vi "Load_Info.vi"(8 "error in (no error)":errorcluster, 11 "AB_RESTfulWebService in":refnum<class "AB_RESTfulWebService.lvclass">) -> (0 "error out":errorcluster, 3 "AB_RESTfulWebService out":refnum<class "AB_RESTfulWebService.lvclass">)   [LabVIEW 2020, in "AB_RESTfulWebService.lvclass"]
uses:
  <vilib>/AppBuilder/AB_Classes/RESTful/AB_RESTfulWebService.lvclass
  e:/builds/penguin/labview/branches/2020/dev/dist/vi.lib/AppBuilder/AB_Classes/Build/AB_Build.lvclass
  <vilib>/AppBuilder/AB_Classes/RESTful/AB_RESTfulWebService.ctl
  <vilib>/AppBuilder/AB_Classes/RESTful/AB_RESTful_RoutingTemplate.ctl
  <vilib>/AppBuilder/AB_Classes/RESTful/AB_RESTful_RoutingType.ctl
  <vilib>/AppBuilder/AB_Classes/RESTful/AB_RESTful_HTTPMethodType.ctl
  <vilib>/AppBuilder/AB_Classes/RESTful/AB_RESTful_ServiceAttribute.ctl
  <vilib>/AppBuilder/AB_Classes/RESTful/AB_RESTful_ServiceAttributeType.ctl
  <vilib>/AppBuilder/RW_Project/AB_RW_Project_PropBag_Action.ctl
  <vilib>/AppBuilder/AB_Classes/RESTful/AB_RESTfulWebService.lvclass/AB_RESTfulWebService.ctl
  <vilib>/AppBuilder/AB_Classes/WebService/AB_WebService.lvclass
  <vilib>/AppBuilder/AB_Classes/Build/AB_Build.lvclass
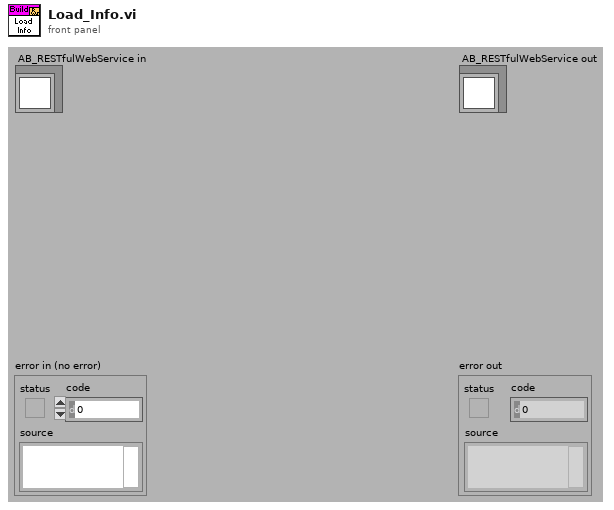
[diagram p1: front panel]
types:
  T1 = typedef "AB_RESTfulWebService.ctl" = cluster{"routing templates":T2[], "defaultStaticDoc":string, "eng_attributes":T5[], "Privilege Mapping":cluster{"Privilege":string, "Description":string, "Role":string}[]}
  T2 = typedef "AB_RESTful_RoutingTemplate.ctl" = cluster{"Template":string, "Routing Type":T3, "HTTP Method Type":T4, "VIName":string, "Default String":string, "Require API key":bool, "Auth permissions":string[], "eng_Static Alias":string, "Required Privilege":string}
  T3 = typedef "AB_RESTful_RoutingType.ctl" = enum32{"Method", "Static"}
  T4 = typedef "AB_RESTful_HTTPMethodType.ctl" = enum32{"GET", "POST", "PUT", "DELETE"}
  T5 = typedef "AB_RESTful_ServiceAttribute.ctl" = cluster{"Name":string, "Service Attribute Type":T6, "Value":string}
  T6 = typedef "AB_RESTful_ServiceAttributeType.ctl" = enum32{"String", "Path"}
  T7 = typedef "AB_RW_Project_PropBag_Action.ctl" = enum16{"read", "write", "clear", "readPrevious", "writePrevious", "clearPrevious"}
  T8 = typedef "AB_Build.ctl" = cluster{"buildSpecName":string, "buildSpecDescription":string, "destinations":refnum<class "AB_Destination.lvclass">[], "exclusionOption":T9, "defaultLanguage":string, "supportedLanguages":string[], "excludedDirectories":path[], "buildContext":refnum<vi>, "buildObject":T10, "preview":bool, "programatic":bool, "progressBarEvents":T11, "userLog_Path":path, "preActionID":string, "preAction_Path":path, "postActionID":string, "postAction_Path":path, "eng_checkForBrokenVIs?":bool, "eng_verboseLinkerErrors?":bool, "localDest_Path":path, "targetDest_Path":path, "removeVIObject":u16, "cache":refnum<class "PreviewCache.lvclass">, "use cache":bool, "previewCache_ID":string, "buildCache_ID":string, "eng_TempLocalDest_Path":path, "eng_collectDependencies?":bool, "versionInfo":cluster{"buildVersion":cluster{"major":u16, "minor":u16, "patch":u16, "build":u16}, "autoIncrement":bool}, "eng_enableVIChecksums":bool}
  T9 = typedef "AB_Exclusion_Option.ctl" = cluster{"typedefs":bool, "polymorphicVIs":bool, "unusedLibraryItems":bool, "modifyLibraryFile":bool, "edit-timeDependencies":bool, "inlineVIs":bool, "dependent PPLs":bool, "dependent DLLs":bool}
  T10 = typedef "ItemRef.ctl" = u64
  T11 = typedef "provcom_ProgressBar_Events.ctl" = cluster{"newJob":refnum<user-event>, "newItem":refnum<user-event>, "errorMsg":T12, "cancel":refnum<user-event>}
  T12 = typedef "mxLvBuildError.ctl" = refnum<user-event>
  T13 = typedef "AB_RW_Project_RESTfulWebService_Data.ctl" = cluster{"routing templates":T14[], "defaultStaticDoc":string}
  T14 = typedef "AB_RW_Project_RESTful_RoutingTemplate.ctl" = cluster{"Template":string, "Routing Type":T3, "HTTP Method Type":T4, "VIName":string, "Default String":string, "Require API key":bool, "Auth permissions":string}
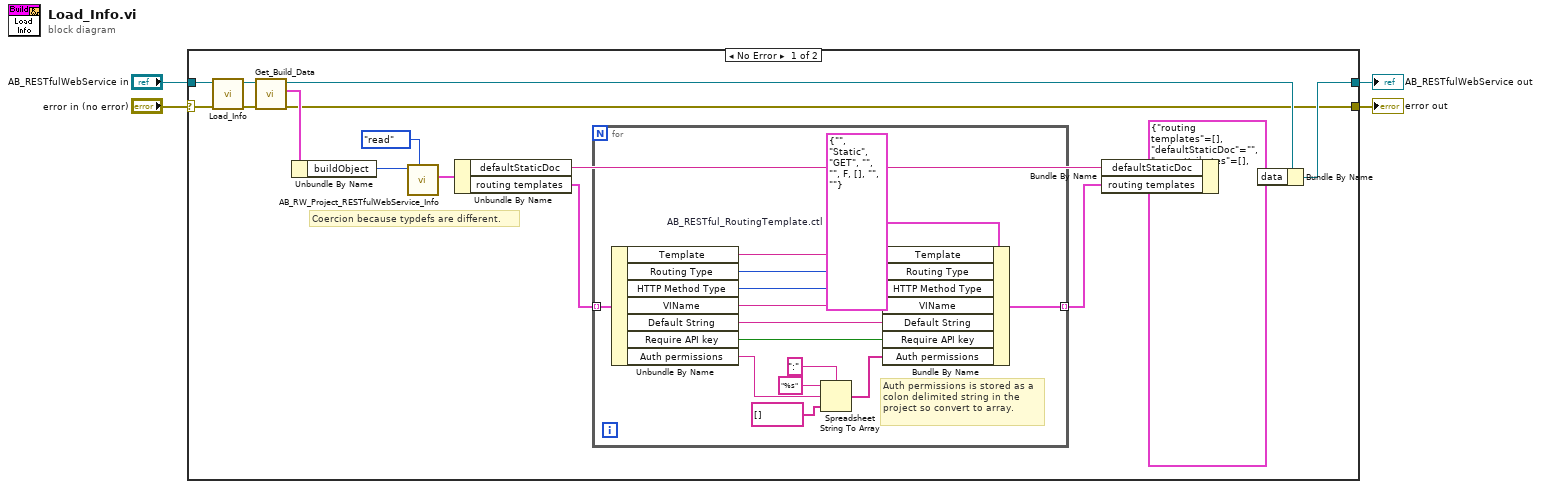
[diagram p0: block diagram]
diagram:
  n1 = case shown="No Error" "error in (no error)" {
    selector: "error in (no error)" -> [w19 w35]
    tunnel: [w11 w35] -> w4
    tunnel: [w12 w36] -> w3
    tunnel: "AB_RESTfulWebService in" -> [w20 w36]
    frame No Error {
      # "Coercion because typdefs are different."
      n2 = call-parent "Load_Info.vi"("error in (no error)"=w19, "AB_WebService in"=w20) -> ("error out"=w13:errorcluster, "AB_WebService out"=w14:refnum<class "AB_RESTfulWebService.lvclass">)  [unwired: 8 in]
      n3 = call <vilib>:"Get_Build_Data.vi"("error in (no error)"=w13, "Class in"=w14) -> ("error out"=w11:errorcluster, "data"=w15:T8, "Class out"=w16:refnum<class "AB_RESTfulWebService.lvclass">)  [unwired: 7 in]
      n4 = Unbundle By Name(w15) -> ("buildObject"=w17:T10)
      n5 = call <vilib>:"AB_RW_Project_RESTfulWebService_Info.vi"("action"=AB_RW_Project_PropBag_Action."read", "Object In"=w17) -> ("RESTfulWebServiceInfo out"=w10:T13)  [unwired: 7 in, 2 out]
      n6 = Unbundle By Name(w10) -> ("defaultStaticDoc"=w7:string, "routing templates"=w6:T14[])
      n7 = for {
        tunnel: w6 -> [w34] mode=indexing
        tunnel: [w21] -> w5 mode=indexing
        w29 = T2 {"Template"="", "Routing Type"=enum."Static", "HTTP Method Type"=enum."GET", "VIName"="", "Default String"="", "Require API key"=FALSE, "Auth permissions"=[], "eng_Static Alias"="", "Required Privilege"=""}  # AB_RESTful_RoutingTemplate.ctl
        # "Auth permissions is stored as a colon delimited string in the project so convert to array."
        n8 = Unbundle By Name(w34) -> ("Template"=w28:string, "Routing Type"=w27:T3, "HTTP Method Type"=w26:T4, "VIName"=w25:string, "Default String"=w23:string, "Require API key"=w24:bool, "Auth permissions"=w30:string)
        n9 = Spreadsheet String To Array(delimiter (Tab)=":", format string="%s", spreadsheet string=w30, array type (2D Dbl)=string[] [] ("web servers")) -> (array=w22:string[])
        n10 = Bundle By Name(cluster=w29, "Template"=w28, "Routing Type"=w27, "HTTP Method Type"=w26, "VIName"=w25, "Default String"=w23, "Require API key"=w24, "Auth permissions"=w22) -> (w21:T2)
      }
      n11 = Bundle By Name(cluster=T1 {"routing templates"=[], "defaultStaticDoc"="", "eng_attributes"=[], "Privilege Mapping"=[]} ("data"), "defaultStaticDoc"=w7, "routing templates"=w5) -> (w8:T1)
      n12 = Bundle By Name(cluster=w16, "data"=w8) -> (w12:refnum<class "AB_RESTfulWebService.lvclass">)
    }
    frame Error {
    }
  }
  "error out" <- w4
  "AB_RESTfulWebService out" <- w3
